vi "Set Destination Preserve Hierarchy.vi"(8 "error in (no error)":errorcluster, 9 "Preserve Hierarchy":bool, 10 "Destination label":string, 11 "Build in":refnum<class "NI_AB_API_Build.lvclass">) -> (0 "error out":errorcluster, 3 "Build out":refnum<class "NI_AB_API_Build.lvclass">)   [LabVIEW 2020, in "NI_AB_API_Build.lvclass"]
uses:
  <vilib>/AppBuilder/AB_API/Build/NI_AB_API_Build.lvclass
  <vilib>/AppBuilder/AB_API/Build/NI_AB_API_Build.lvclass/NI_AB_API_Build.ctl
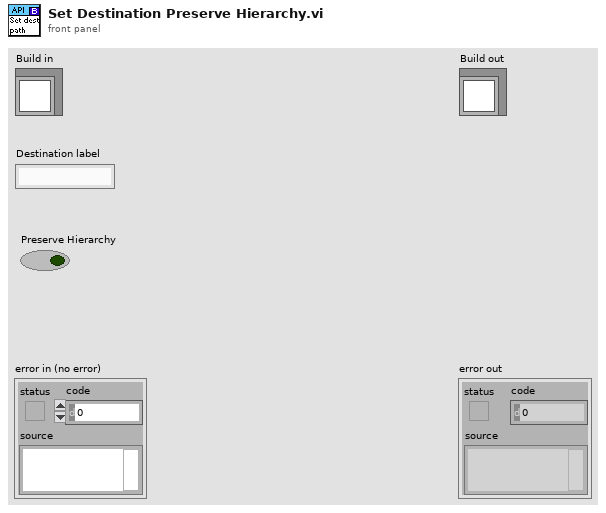
[diagram p1: front panel]
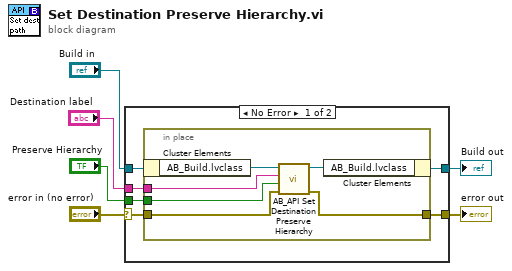
[diagram p0: block diagram]
diagram:
  n1 = case shown="No Error" "error in (no error)" {
    selector: "error in (no error)" -> [w10 w20]
    tunnel: [w7 w20] -> w5
    tunnel: [w8 w19] -> w3
    tunnel: "Build in" -> [w9 w19]
    tunnel: "Destination label" -> [w12 _]
    tunnel: "Preserve Hierarchy" -> [w11 _]
    frame No Error {
      n2 = in-place {
        in-place-border: w12 -> [w14]
        in-place-border: w11 -> [w13]
        in-place-border: w10 -> [w15]
        in-place-border: [w16] -> w7
        n3 = in-place-cluster #1(w9) -> ("AB_Build.lvclass"=w18:refnum<class "AB_Build.lvclass">)
        n4 = call <vilib>:"AB_API Set Destination Preserve Hierarchy.vi"("error in (no error)"=w15, "Preserve Hierarchy"=w13, "Destination label"=w14, "Build in"=w18) -> ("error out"=w16:errorcluster, "Build out"=w17:refnum<class "AB_Build.lvclass">)  [unwired: 6 in]
        n5 = in-place-cluster #1("AB_Build.lvclass"=w17) -> (w8:refnum<class "NI_AB_API_Build.lvclass">)
      }
    }
    frame Error {
    }
  }
  "error out" <- w5
  "Build out" <- w3
